vi "Connect Channels.vi"(8 "error in (no error)":errorcluster, 9 "instance id":string, 10 "Maps":T1[](array[typedef]), 11 "Engine Configuration in":refnum<class "engine configuration.lvclass">) -> (0 "error out":errorcluster, 3 "Engine Configuration out":refnum<class "engine configuration.lvclass">)   [LabVIEW 2015, in "Sequencer Module editor node.lvclass"]
doc: "Creates mappings or connections between Tags and Channels according to the data in the 'Maps' input."
uses:
  Sequencer Module editor node.lvclass
  Map.ctl
  <vilib>/NI/Tag Bus Module Framework/channel/TBM channel.lvclass
  <vilib>/NI/Module Execution Interface/Engine Configuration/engine configuration.lvclass
  <vilib>/NI/Tag Bus/tag/tag descriptor.lvclass/tag descriptor.ctl
  <vilib>/NI/Tag Bus/tag/write tag name.vi
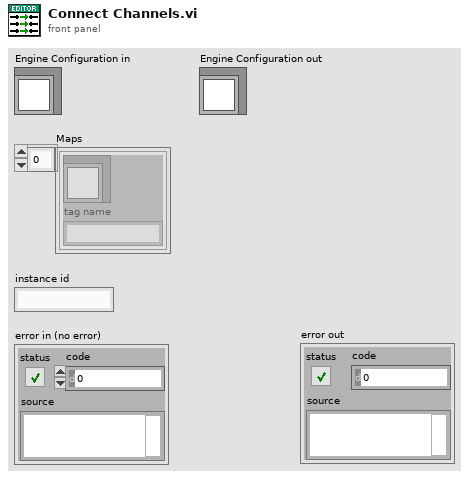
[diagram p1: front panel]
types:
  T1 = typedef "Sequencer Module editor node.lvclass/Map.ctl" = cluster{"channel":refnum<class "TBM channel.lvclass">, "tag name":string}
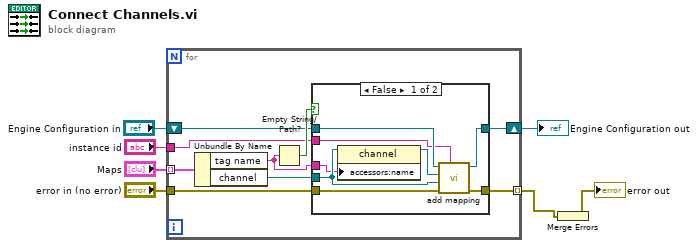
[diagram p0: block diagram]
diagram:
  n1 = for {
    tunnel: "error in (no error)" -> [w15]
    tunnel: [w13] -> w2 mode=indexing
    tunnel: "instance id" -> [w11]
    tunnel: "Maps" -> [w10] mode=indexing
    shift-right: [w14] -> w4
    shift-left: "Engine Configuration in" -> [w12]
    n2 = Unbundle By Name(w10) -> ("tag name"=w9:string, "channel"=w8:refnum<class "TBM channel.lvclass">)
    n3 = Empty String/Path?(string/path=w9) -> (empty?=w16:bool)
    n4 = case shown="False" w16 {
      tunnel: w12 -> [w24 w26]
      tunnel: [w23 w26] -> w14
      tunnel: w8 -> [w22 _]
      tunnel: w9 -> [w21 _]
      tunnel: [w19 w25] -> w13
      tunnel: w15 -> [w18 w25]
      tunnel: w11 -> [w17 _]
      frame False {
        n5 = property class="channel"(reference=w22, "accessors:name"=w21) -> (reference out=w20:refnum<class "TBM channel.lvclass">)  [unwired: 1 in, 1 out]
        n6 = call-dynamic "add mapping.vi"("owner ID"=w17, "error in"=w18, "channel"=w22, "tag descriptor"=w20, "engine configuration"=w24) -> ("error out"=w19:errorcluster, "engine configuration out"=w23:refnum<class "engine configuration.lvclass">)  [unwired: 5 in]
      }
      frame True {
      }
    }
  }
  "Engine Configuration out" <- w4
  n7 = Merge Errors(w2) -> (→"error out":errorcluster)
